vi "read_settings_file.vi"(8 "error in (no error)":errorcluster, 10 "settings name":string, 11 "GenericComponent in":refnum<class "GenericComponent.lvclass">) -> (0 "error out":errorcluster, 1 "cancelled?":bool, 2 "settings cluster out":variant, 3 "GenericComponent out":refnum<class "GenericComponent.lvclass">, 4 "settings name":string)   [LabVIEW 2010, in "GenericComponent.lvclass"]
uses:
  GenericComponent.lvclass
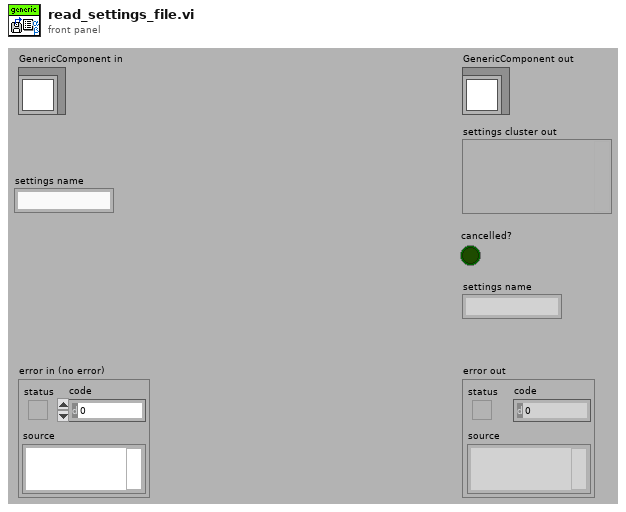
[diagram p1: front panel]
types:
  T1 = enum16{"open", "replace", "create", "open or create", "replace or create", "replace or create with confirmation"}
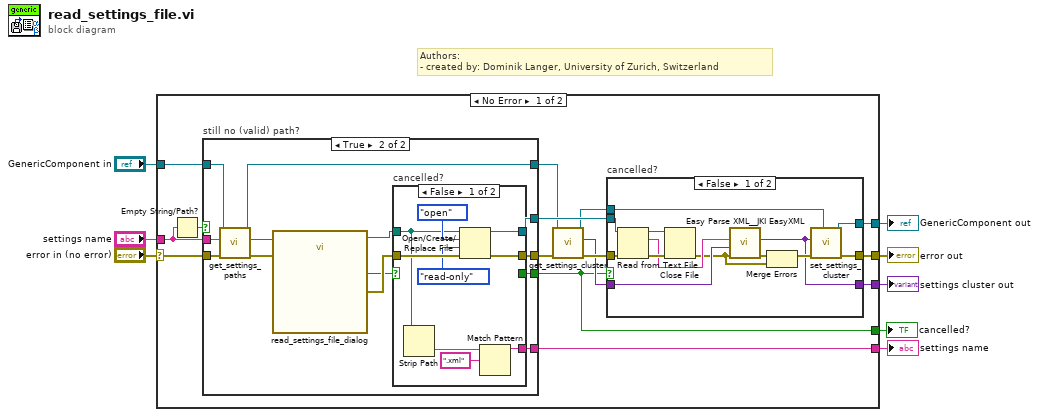
[diagram p0: block diagram]
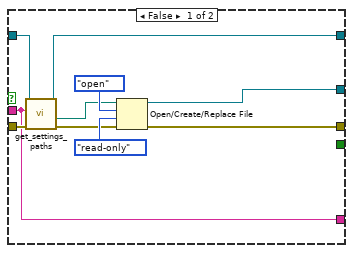
[diagram p3: hidden frame]
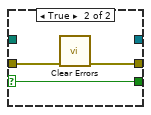
[diagram p4: hidden frame]
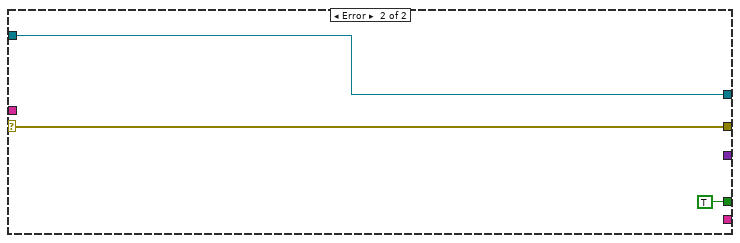
[diagram p5: hidden frame]
diagram:
  # "Authors: \n- created by: Dominik Langer, University of Zurich, Switzerland"
  n1 = case shown="No Error" "error in (no error)" {
    selector: "error in (no error)" -> [w22 w77]
    tunnel: [w17 w77] -> w7
    tunnel: [w19 w76] -> w5
    tunnel: "GenericComponent in" -> [w21 w76]
    tunnel: "settings name" -> [w23 _]
    tunnel: [w18 _] -> w3
    tunnel: [w10 TRUE] -> w2
    tunnel: [w9 _] -> w1
    frame No Error {
      n2 = Empty String/Path?(string/path=w23) -> (empty?=w20:bool)
      n3 = case "still no (valid) path?" shown="True" w20 {
        tunnel: w23 -> [w40 w62]
        tunnel: w22 -> [w49 w61]
        tunnel: w21 -> [w41 w60]
        tunnel: [w42 w59] -> w14
        tunnel: [w44 w55] -> w12
        tunnel: [w43 w52] -> w16
        tunnel: [_ w51] -> w10
        tunnel: [w40 w50] -> w9
        frame False {
          n4 = call-dynamic "get_settings_paths.vi"("error in (no error)"=w49, "file name"=w40, "GenericComponent in"=w41) -> ("error out"=w46:errorcluster, "settings file path"=w45:path, "GenericComponent out"=w42:refnum<class "GenericComponent.lvclass">)  [unwired: 3 in, 3 out]
          n5 = Open/Create/Replace File(file path (use dialog)=w45, error in=w46, operation (0:open)=T1."open", access (0:read/write)=enum16{"read/write", "read-only", "write-only"}."read-only") -> (refnum out=w43:refnum<file>, error out=w44:errorcluster)  [unwired: 2 in, 1 out]
        }
        frame True {
          n6 = call-dynamic "get_settings_paths.vi"("error in (no error)"=w61, "file name"=w62, "GenericComponent in"=w60) -> ("error out"=w58:errorcluster, "settings folder for a specific component"=w57:path, "GenericComponent out"=w59:refnum<class "GenericComponent.lvclass">)  [unwired: 3 in, 3 out]
          n7 = call "read_settings_file_dialog.vi"("start path"=w57, "error in"=w58) -> ("selected path"=w56:path, "cancelled"=w53:bool, "error out"=w54:errorcluster)  [unwired: 10 in, 1 out]
          n8 = case "cancelled?" shown="False" w53 {
            selector: w53 -> [_ w72]
            tunnel: w56 -> [w66 _]
            tunnel: [w71 w73] -> w55
            tunnel: w54 -> [w70 w74]
            tunnel: [w67 _] -> w52
            tunnel: [_ w72] -> w51
            tunnel: [w65 _] -> w50
            frame False {
              n9 = Strip Path(path=w66) -> (name=w64:string)  [unwired: 1 out]
              n10 = Open/Create/Replace File(file path (use dialog)=w66, error in=w70, operation (0:open)=T1."open", access (0:read/write)=enum16{"read/write", "read-only", "write-only"}."read-only") -> (refnum out=w67:refnum<file>, error out=w71:errorcluster)  [unwired: 2 in, 1 out]
              n11 = Match Pattern(string=w64, regular expression=".xml") -> (before substring=w65:string)  [unwired: 1 in, 3 out]
            }
            frame True {
              n12 = call <vilib>:"Clear Errors.vi"("error in (no error)"=w74) -> ("error out"=w73:errorcluster)  [unwired: 6 in]
            }
          }
        }
      }
      n13 = call-dynamic "get_settings_cluster.vi"("error in (no error)"=w12, "GenericPlugin in"=w14) -> ("error out"=w13:errorcluster, "settings cluster"=w11:variant, "GenericPlugin out"=w15:refnum<class "GenericComponent.lvclass">)  [unwired: 7 in]
      n14 = case "cancelled?" shown="False" w10 {
        tunnel: w13 -> [w36 w38]
        tunnel: w15 -> [w25 w37]
        tunnel: [w28 w37] -> w19
        tunnel: [w24 w39] -> w18
        tunnel: [w29 w38] -> w17
        tunnel: w16 -> [w34 _]
        tunnel: w11 -> [w27 w39]
        frame False {
          n15 = Read from Text File(file (use dialog)=w34, error in=w36) -> (refnum out=w33:refnum<file>, text=w32:string, error out=w35:errorcluster)  [unwired: 2 in, 1 out]
          n16 = Close File(refnum=w33, error in=w35) -> (error out=w26:errorcluster)  [unwired: 1 out]
          n17 = call <vilib>:"Easy Parse XML__JKI EasyXML.vi"("error in (no error)"=w26, "LabVIEW Data (Type)"=w27, "XML String"=w32) -> ("error out"=w31:errorcluster, "LabVIEW Data"=w24:variant)  [unwired: 7 in]
          n18 = Merge Errors(w31, w26) -> (w30:errorcluster)
          n19 = call-dynamic "set_settings_cluster.vi"("error in (no error)"=w30, "settings cluster variant"=w24, "GenericComponent in"=w25) -> ("error out"=w29:errorcluster, "GenericComponent out"=w28:refnum<class "GenericComponent.lvclass">)  [unwired: 7 in]
        }
        frame True {
        }
      }
    }
    frame Error {
    }
  }
  "error out" <- w7
  "GenericComponent out" <- w5
  "settings cluster out" <- w3
  "cancelled?" <- w2
  "settings name" <- w1
